vi "例4.7 循环结构内外数据的交换举例.vi"() -> ()   [LabVIEW 2017]
panel:
  out "乘积2":dbl
  out "乘积1":dbl
  in  "y":dbl
  in  "x":dbl
  in  "停止":bool
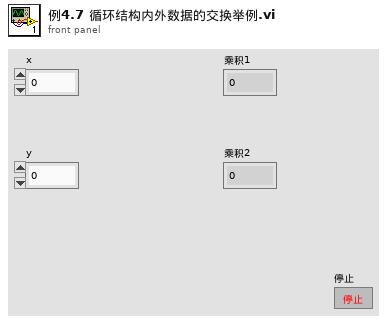
[diagram p1: front panel]
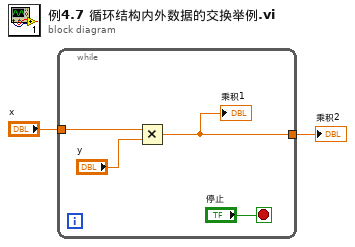
[diagram p0: block diagram]
diagram:
  n1 = while {
    tunnel: "x" -> [w5]
    tunnel: [w3] -> w1
    stop <- "停止" stop-if-true
    n2 = Multiply(x=w5, y="y") -> (x*y=w3:dbl)
    "乘积1" <- w3
  }
  "乘积2" <- w1
